vi "writeU16FIFO.vi"(8 "error in (no error)":errorcluster, 9 "Timeout":i32, 10 "Data":u16[](array[numeric]), 11 "ModbusSubnetBTxDataFIFO in":refnum<class "ModbusSubnetBTxDataFIFO.lvclass">) -> (0 "error out":errorcluster, 2 "ElementsRemaining":u32, 3 "ModbusSubnetBTxDataFIFO out":refnum<class "ModbusSubnetBTxDataFIFO.lvclass">)   [LabVIEW 2016, in "ModbusSubnetBTxDataFIFO.lvclass"]
uses:
  ModbusSubnetBTxDataFIFO.lvclass
  ModbusSubnetBTxDataFIFO.lvclass/ModbusSubnetBTxDataFIFO.ctl
  FPGA/FPGA.lvclass
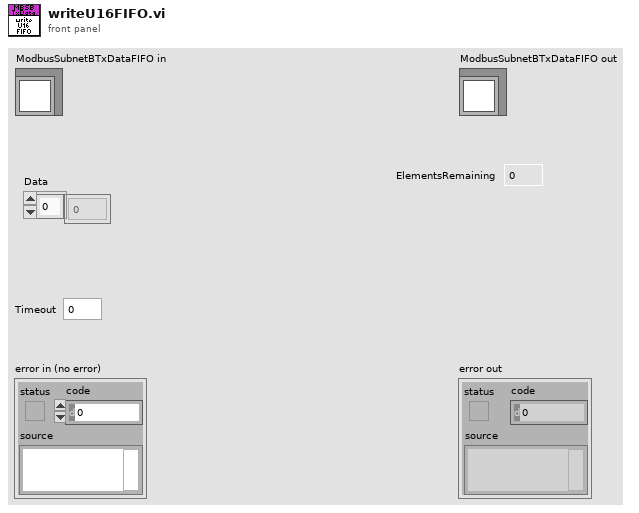
[diagram p1: front panel]
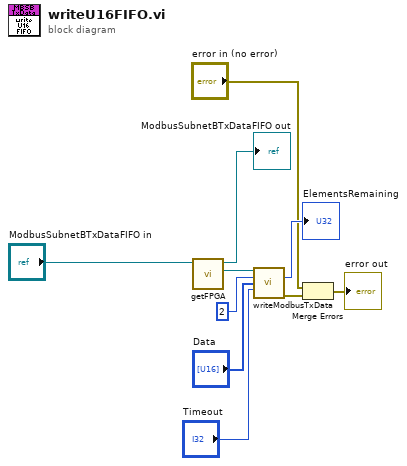
[diagram p0: block diagram]
diagram:
  n1 = call "getFPGA.vi"("ModbusSubnetBTxDataFIFO in"="ModbusSubnetBTxDataFIFO in") -> ("FPGA"=w9:refnum<class "FPGA.lvclass">, "ModbusSubnetBTxDataFIFO out"=→"ModbusSubnetBTxDataFIFO out":refnum<class "ModbusSubnetBTxDataFIFO.lvclass">)  [unwired: 9 in]
  n2 = call "writeModbusTxData.vi"("FPGA in"=w9, "Subnet"=u16 2, "Data"="Data", "Timeout (ms)"="Timeout") -> ("Empty Elements Remaining"=→"ElementsRemaining":u32, "error out"=w3:errorcluster)  [unwired: 9 in, 1 out]
  n3 = Merge Errors("error in (no error)", w3) -> (→"error out":errorcluster)
